vi "TriggeredAcqDemo-Config.vi"(10 "Npts":i32=25000, 11 "Fs":dbl=100000.0 format="%#_13g") -> (0 "error out":errorcluster, 3 "tasks":refnum<k21>[](array[refnum]))   [LabVIEW 2015]
uses:
  <vilib>/DAQmx/create/channels.llb/DAQmx Create Channel (AO-Voltage-Basic).vi
  <vilib>/DAQmx/create/channels.llb/DAQmx Create Channel (AI-Voltage-Basic).vi
  <vilib>/DAQmx/configure/timing.llb/DAQmx Timing (Sample Clock).vi
  <vilib>/DAQmx/configure/trigger.llb/DAQmx Start Trigger (Digital Edge).vi
  <resource>/objmgr/daqmx.rc
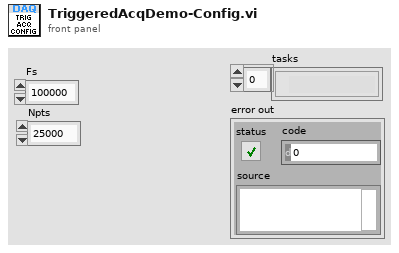
[diagram p1: front panel]
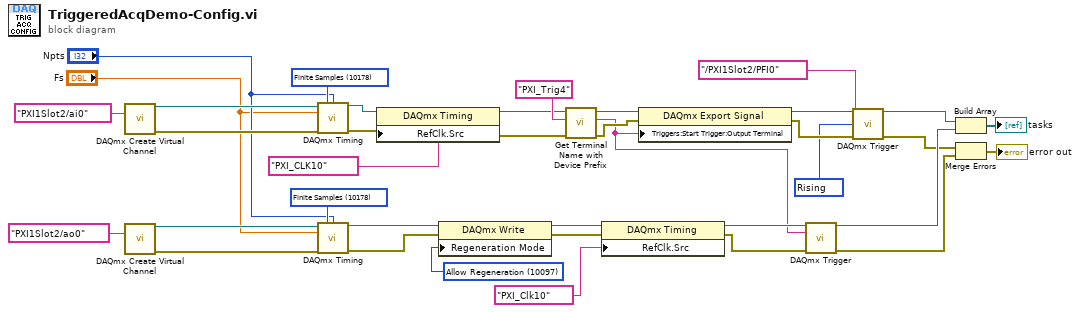
[diagram p0: block diagram]
diagram:
  w2 = 10280 items=["Rising"=10280, "Falling"=10171] ("edge")
  w28 = 10178 items=["Finite Samples"=10178, "Continuous Samples"=10123, "Hardware Timed Single Point"=12522] ("sample mode")
  w31 = 10097 items=["Allow Regeneration"=10097, "Do Not Allow Regeneration"=10158] ("RegenMode")
  w35 = 10178 items=["Finite Samples"=10178, "Continuous Samples"=10123, "Hardware Timed Single Point"=12522] ("sample mode")
  n1 = call-poly <vilib>:"DAQmx Create Virtual Channel.vi"("physical channels"=tag "PXI1Slot2/ai0") -> ("task out"=w37:refnum<k21>, "error out"=w36:errorcluster)  [unwired: 13 in]
  n2 = call-poly <vilib>:"DAQmx Create Virtual Channel.vi"("physical channels"=tag "PXI1Slot2/ao0") -> ("task out"=w34:refnum<k21>, "error out"=w30:errorcluster)  [unwired: 13 in]
  n3 = call-poly <vilib>:"DAQmx Timing.vi"("task/channels in"=w37, "sample mode"=w35, "samples per channel"="Npts", "rate"="Fs", "error in"=w36) -> ("task out"=w17:refnum<k21>, "error out"=w16:errorcluster)  [unwired: 9 in]
  n4 = call-poly <vilib>:"DAQmx Timing.vi"("task/channels in"=w34, "sample mode"=w28, "samples per channel"="Npts", "rate"="Fs", "error in"=w30) -> ("task out"=w32:refnum<k21>, "error out"=w33:errorcluster)  [unwired: 9 in]
  n5 = property class="DAQmx Timing"(reference=w17, error in=w16, "RefClk.Src"=tag "PXI_CLK10") -> (reference out=w12:refnum<k21>, error out=w11:errorcluster)
  n6 = property class="DAQmx Write"(reference=w32, error in=w33, "Regeneration Mode"=w31) -> (reference out=w27:refnum<k21>, error out=w26:errorcluster)
  n7 = call "Get Terminal Name with Device Prefix.vi"("error in (no error)"=w11, "Local Terminal Name"="PXI_Trig4", "task/channels in"=w12) -> ("error out"=w22:errorcluster, "Terminal Name with Device Prefix"=w13:tag, "task out"=w21:refnum<k21>)  [unwired: 6 in]
  n8 = property class="DAQmx Timing"(reference=w27, error in=w26, "RefClk.Src"=tag "PXI_Clk10") -> (reference out=w20:refnum<k21>, error out=w19:errorcluster)
  n9 = property class="DAQmx Export Signal"(reference=w21, error in=w22, "Triggers:Start Trigger:Output Terminal"=w13) -> (reference out=w6:refnum<k21>, error out=w5:errorcluster)
  n10 = call-poly <vilib>:"DAQmx Trigger.vi"("task/channels in"=w20, "source"=w13, "error in"=w19) -> ("task out"=w8:refnum<k21>, "error out"=w7:errorcluster)  [unwired: 11 in]
  n11 = call-poly <vilib>:"DAQmx Trigger.vi"("task/channels in"=w6, "source"=tag "/PXI1Slot2/PFI0", "edge"=w2, "error in"=w5) -> ("task out"=w4:refnum<k21>, "error out"=w3:errorcluster)  [unwired: 10 in]
  n12 = Build Array(w4, w8) -> (→"tasks":refnum<k21>[])
  n13 = Merge Errors(w3, w7) -> (→"error out":errorcluster)
